vi "Calculate Scan Spots (SubVI).vi"(1 "Start Location (Pixels)":cluster{"X":i32, "Y":i32}={"X"=200, "Y"=200}, 2 "End Location (Pixels)":cluster{"X":i32, "Y":i32}={"X"=2800, "Y"=2800}, 3 "STEP Size (Pixels)":i32=400) -> (4 "Scan Spots (Array)":cluster{"X":i32, "Y":i32}[](array[cluster]), 15 "Spot Count":i32[](array[numeric]))   [LabVIEW 2017]
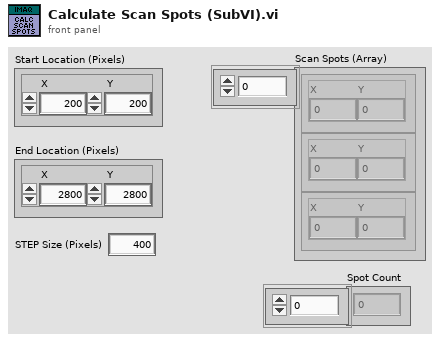
[diagram p1: front panel]
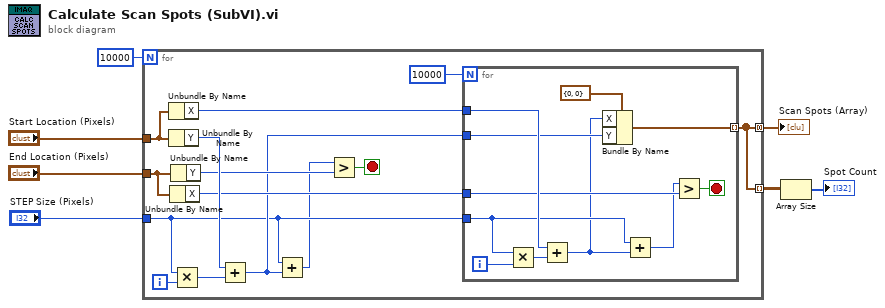
[diagram p0: block diagram]
diagram:
  n1 = for {
    N: 10000 -> [_]
    tunnel: "Start Location (Pixels)" -> [w17]
    tunnel: "End Location (Pixels)" -> [w13]
    tunnel: "STEP Size (Pixels)" -> [w10]
    tunnel: [w8] -> w7 mode=concatenating
    tunnel: [w8] -> w2 mode=indexing
    i -> [w21]
    stop <- w15 stop-if-true
    n2 = Unbundle By Name(w17) -> ("X"=w16:i32)
    n3 = Unbundle By Name(w17) -> ("Y"=w19:i32)
    n4 = Unbundle By Name(w13) -> ("X"=w12:i32)
    n5 = Unbundle By Name(w13) -> ("Y"=w18:i32)
    n6 = Multiply(x=w10, y=w21) -> (x*y=w20:i32)
    n7 = Add(x=w19, y=w20) -> (x+y=w11:i32)
    n8 = Add(x=w10, y=w11) -> (x+y=w9:i32)
    n9 = Greater?(x=w9, y=w18) -> (0:w15:bool)
    n10 = for {
      N: 10000 -> [_]
      tunnel: w10 -> [w24]
      tunnel: w16 -> [w30]
      tunnel: w12 -> [w29]
      tunnel: w11 -> [w26]
      tunnel: [w25] -> w8 mode=indexing
      i -> [w31]
      stop <- w28 stop-if-true
      n11 = Multiply(x=w24, y=w31) -> (x*y=w32:i32)
      n12 = Add(x=w30, y=w32) -> (x+y=w23:i32)
      n13 = Bundle By Name(cluster=cluster{"X":i32, "Y":i32} {"X"=0, "Y"=0} ("Start Location (Pixels)"), "X"=w23, "Y"=w26) -> (w25:cluster{"X":i32, "Y":i32})
      n14 = Add(x=w24, y=w23) -> (x+y=w22:i32)
      n15 = Greater?(x=w22, y=w29) -> (0:w28:bool)
    }
  }
  "Scan Spots (Array)" <- w7
  n16 = Array Size(array=w2) -> (size(s)=→"Spot Count":i32[])
